vi "读取connection reference.vi"(8 "error in (no error)":errorcluster caption="错误输入（无错误）", 11 "database输入":refnum<class "database.lvclass">) -> (0 "error out":errorcluster caption="错误输出", 2 "reference":T1, 3 "database输出":refnum<class "database.lvclass">)   [LabVIEW 2016, in "中水三立SQL数据传输.lvlib" / "database.lvclass"]
uses:
  database.lvclass
  <vilib>/addons/database/Connection.llb/Conn ObjectReference.ctl
  database.lvclass/database.ctl
  <vilib>/addons/database/NI_Database_API.lvlib
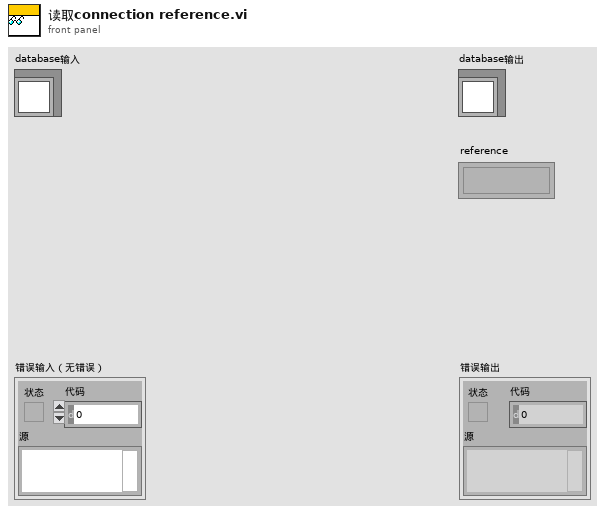
[diagram p1: front panel]
types:
  T1 = typedef "NI_Database_API.lvlib/Conn ObjectReference.ctl" = refnum<k1>
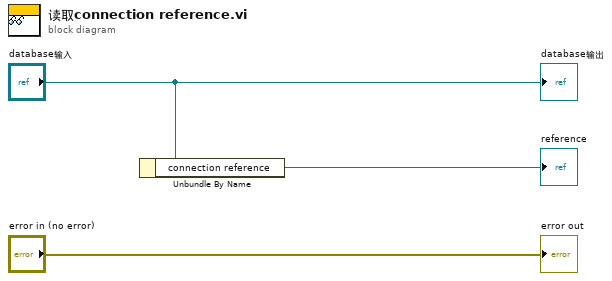
[diagram p0: block diagram]
diagram:
  n1 = Unbundle By Name("database输入") -> ("connection reference"=→"reference":T1)
  "error out" <- "error in (no error)"
  "database输出" <- "database输入"
